vi "Example Interrupt.vi"() -> ()   [LabVIEW 2010]
uses:
  C:/tf/play/labview/Tinkerforge.dll
  Tinkerforge.dll
panel:
  out "value":bool
  out "changed":bool
  out "channel":u8
  in  "stop":bool
  in  "uid":string="xyz"
  in  "port":i32=4223
  in  "host":string="localhost"
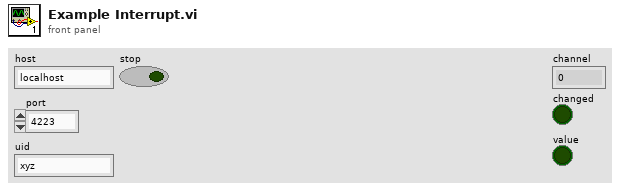
[diagram p1: front panel]
types:
  T1 = cluster{"channel":u8, "changed":bool, "value":bool}
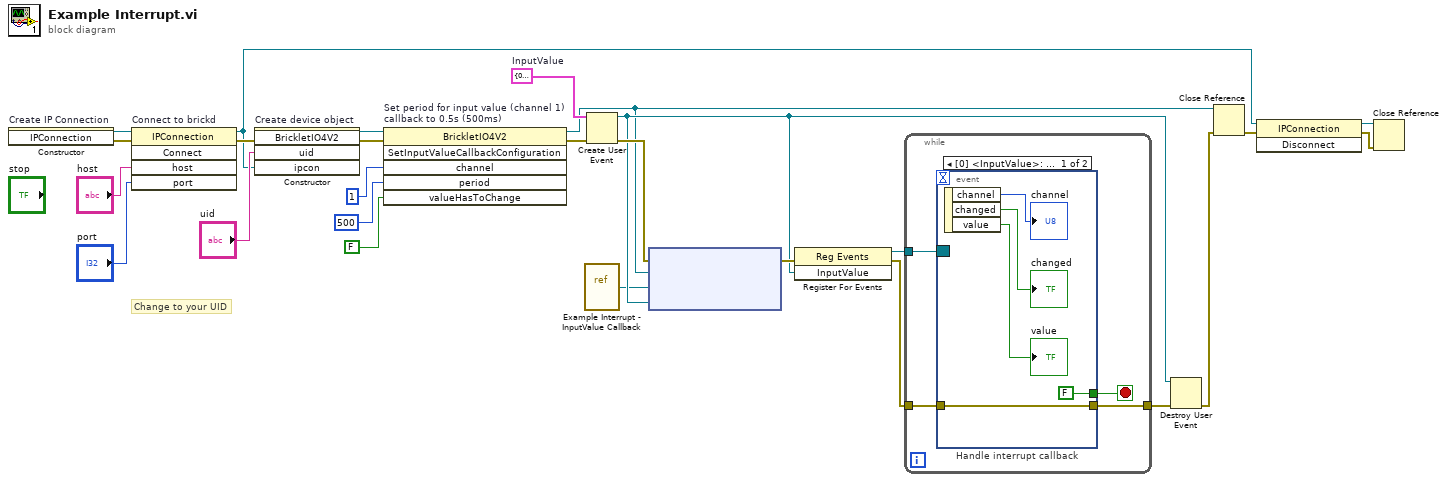
[diagram p0: block diagram]
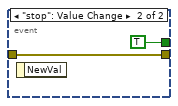
[diagram p2: hidden frame]
diagram:
  w10 = T1 {"channel"=0, "changed"=FALSE, "value"=FALSE}  # InputValue
  # "Change to your UID"
  n1 = constructor on="Create IP Connection" class="IPConnection"() -> (reference out=w26:refnum<k24>, error out=w5:errorcluster)  [unwired: 3 in, 1 out]
  n2 = invoke on="Connect to brickd" class="IPConnection" method="Connect"(reference=w26, error in=w5, "host"="host", "port"="port") -> (reference out=w19:refnum<k24>, error out=w22:errorcluster)  [unwired: 1 in, 3 out]
  n3 = constructor on="Create device object" class="BrickletIO4V2"(error in=w22, "uid"="uid", "ipcon"=w19) -> (reference out=w7:refnum<k24>, error out=w9:errorcluster)  [unwired: 2 in, 3 out]
  n4 = invoke on="Set period for input value (channel 1)\ncallback to 0.5s (500ms)" class="BrickletIO4V2" method="SetInputValueCallbackConfiguration"(reference=w7, error in=w9, "channel"=u8 1, "period"=i64 500, "valueHasToChange"=FALSE) -> (reference out=w6:refnum<k24>, error out=w8:errorcluster)  [unwired: 1 in, 4 out]
  n5 = vi-ref "Example Interrupt - InputValue Callback.vi"() -> ("vi reference"=w1:refnum<vi>)
  n6 = Create User Event(user event datatype=w10, error in=w8) -> (user event=w12:refnum<user-event>, error out=w17:errorcluster)
  n7 = node ("Register Event Callback")(w17, w6, w1, w12) -> (w16:errorcluster)  [unwired: 1 in, 1 out]
  n8 = register-events(error in=w16, w12) -> (reference out=w15:refnum<event-registration>, error out=w13:errorcluster)  [unwired: 1 in]
  n9 = while {
    tunnel: w15 -> [w30]
    tunnel: [w29] -> w14
    tunnel: w13 -> [w28]
    stop <- w27 stop-if-true
    n10 = event "Handle interrupt callback" shown="[0] <InputValue>: User Event" {
      selector: w30 -> [_ _]
      dyn-events: _ -> [_ _]
      timeout: _ -> [_ _]
      tunnel: [w35 w36] -> w29
      tunnel: w28 -> [w35 w36]
      tunnel: [FALSE TRUE] -> w27
      event User Event {
        n11 = event-data() -> ("channel"=→"channel":u8, "changed"=→"changed":bool, "value"=→"value":bool)  [unwired: 1 in]
      }
      event "stop": Value Change {
        n12 = event-data() -> ()  [unwired: 1 in, 1 out]
      }
    }
  }
  n13 = Destroy User Event(user event=w12, error in=w14) -> (error out=w11:errorcluster)
  n14 = Close Reference(reference=w6, error in (no error)=w11) -> (error out=w21:errorcluster)
  n15 = invoke class="IPConnection" method="Disconnect"(reference=w19, error in=w21) -> (reference out=w18:refnum<k24>, error out=w20:errorcluster)  [unwired: 1 in, 1 out]
  n16 = Close Reference(reference=w18, error in (no error)=w20) -> ()  [unwired: 1 out]
